vi "CoolLED_Control_v1.0.vi"(8 "error in":errorcluster) -> (0 "error out":errorcluster)   [LabVIEW 2025]
uses:
  SubVIs/States.ctl
  <vilib>/Instr/_visa.llb/VISA Configure Serial Port (Instr).vi
panel:
  in  "Tab Control":enum32{"Commands", "Expert"}(tab)
  in  "Presets":enum16{"DAPI", "GFP", "RFP", "None", "Multiple"}(ring)=enum."None"
  in  "Store":bool
  in  "Cluster":T1 {"Green-Red" step=1 scale=0.0..100.0; "Blue" step=1 scale=0.0..100.0; "Violet" step=1 scale=0.0..100.0}
  in  "VISA resource name":refnum<visa-resource-name>="COM5"
  out "Current command":string="CSSAXF000BXF000CXF000\r\n"
  in  "Stop":bool
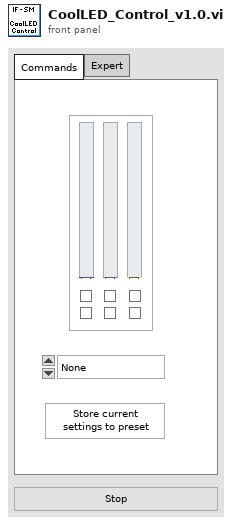
[diagram p1: front panel]
types:
  T1 = cluster{"Violet":u8, "Blue":u8, "Green-Red":u8, "A(S)Selected/(N)Unselected":bool, "B(S)Selected/(N)Unselected":bool, "C(S)Selected/(N)Unselected":bool, "A(N)ON/(F)OFF":bool, "(N)ON/(F)OFF":bool, "C(N)ON/(F)OFF":bool}
  T2 = typedef "States.ctl" = enum16{"Initialize", "Wait for Event", "Close", "Store", "Send", "Create_command", "Presets"}
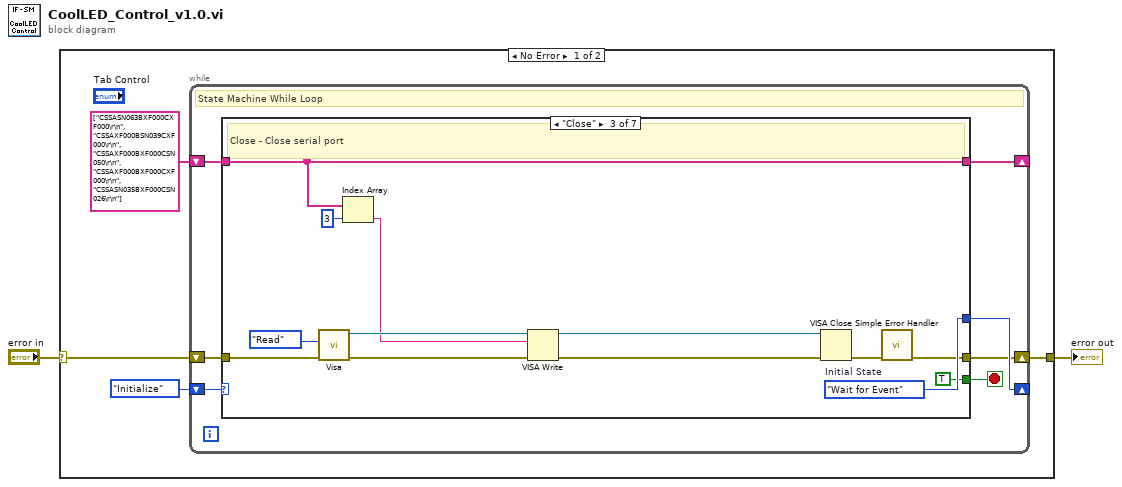
[diagram p0: block diagram]
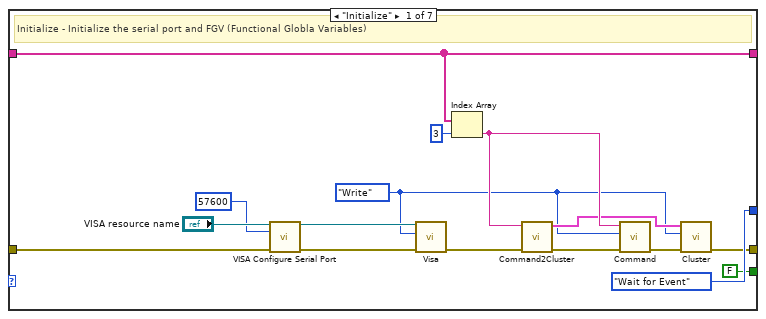
[diagram p2: hidden frame]
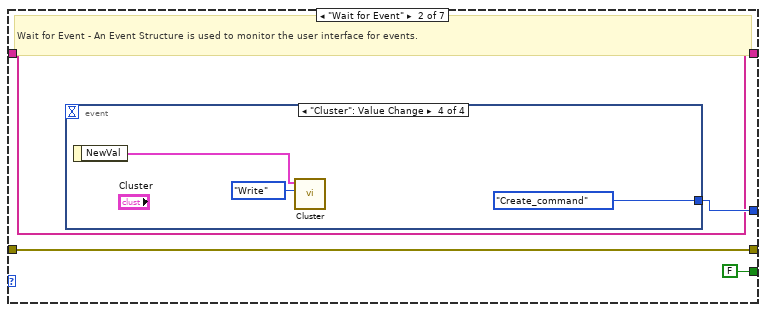
[diagram p3: hidden frame]
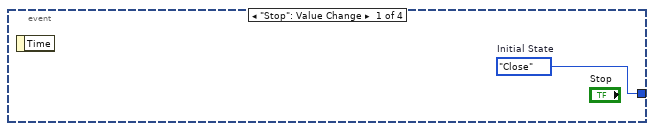
[diagram p4: hidden frame]
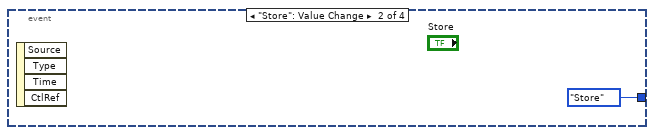
[diagram p5: hidden frame]
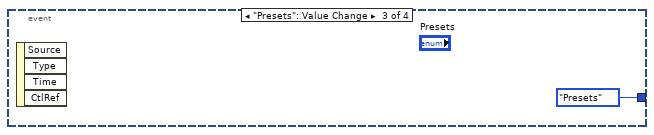
[diagram p6: hidden frame]
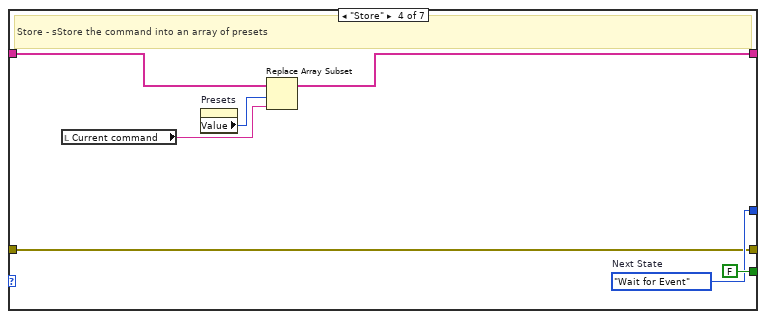
[diagram p7: hidden frame]
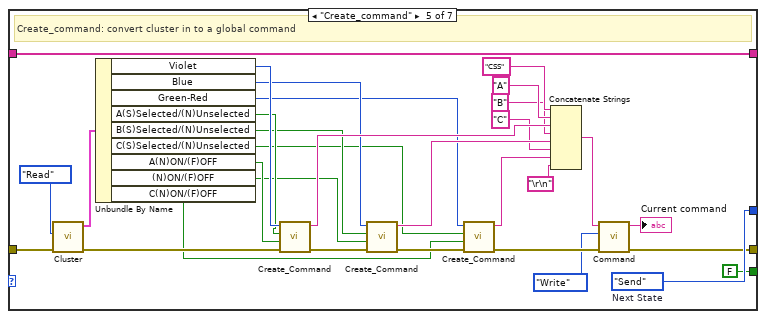
[diagram p8: hidden frame]
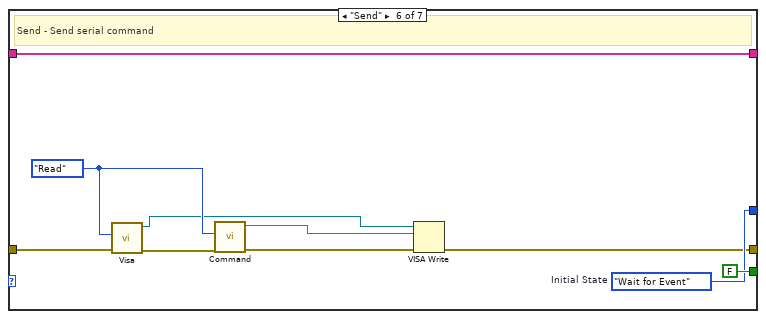
[diagram p9: hidden frame]
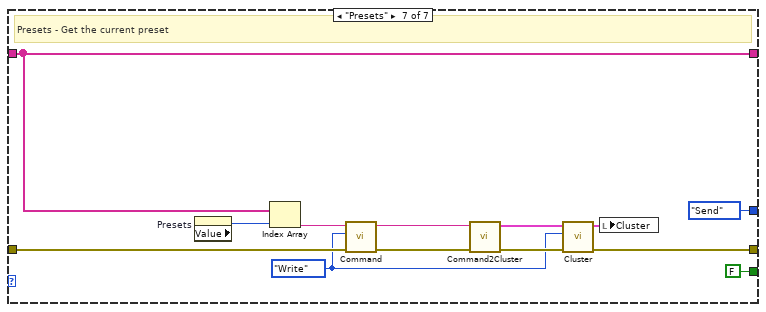
[diagram p10: hidden frame]
diagram:
  n1 = case shown="No Error" "error in" {
    selector: "error in" -> [w5 w114]
    tunnel: [w4 w114] -> w1
    frame No Error {
      n2 = while {
        shift-right: [w13] -> _
        shift-left: States."Initialize" ("Initial State") -> [w11]
        shift-right: [w9] -> w4
        shift-left: w5 -> [w10]
        shift-right: [w7] -> _
        shift-left: string[] ["CSSASN063BXF000CXF000\r\n", "CSSAXF000BSN039CXF000\r\n", "CSSAXF000BXF000CSN050\r\n", "CSSAXF000BXF000CXF000\r\n", "CSSASN035BXF000CSN026\r\n"] ("output array") -> [w8]
        stop <- w12 stop-if-true
        # "State Machine While Loop"
        n3 = case "State Machine Case Structure" shown="\"Close\"" w11 {
          tunnel: [States."Wait for Event" ("Initial State") w33 w52 w58 w90 w99 States."Send" ("Initial State")] -> w13
          tunnel: [FALSE ("Stop the Loop") FALSE ("Stop the Loop") TRUE ("Stop the Loop") FALSE ("Stop the Loop") FALSE ("Stop the Loop") FALSE ("Stop the Loop") FALSE ("Stop the Loop")] -> w12
          tunnel: w10 -> [w26 w31 w47 w57 w72 w94 w110]
          tunnel: [w16 w31 w49 w57 w74 w96 w103] -> w9
          tunnel: w8 -> [w21 w30 w42 w56 w79 w98 w108]
          tunnel: [w21 w30 w42 w53 w79 w98 w108] -> w7
          frame "Initialize" {
            w14 = enum16{"Write", "Read"}."Write" ("Action")
            # "Initialize - Initialize the serial port and FGV (Functional Globla Variables)"
            n4 = call-poly "VISA Configure Serial Port"("VISA resource name"="VISA resource name", "baud rate (9600)"=u32 57600, "error in (no error)"=w26) -> ("VISA resource name out"=w24:refnum<visa-resource-name>, "error out"=w23:errorcluster)  [unwired: 6 in, 5 out]
            n5 = call "Visa.vi"("error in"=w23, "Action"=w14, "VISA resource name"=w24) -> ("error out"=w22:errorcluster)  [unwired: 7 in, 1 out]
            n6 = Index Array(array=w21, index=3) -> (element=w19:string)
            n7 = call "Command2Cluster.vi"("error in"=w22, "Current command"=w19) -> ("error out"=w18:errorcluster, "Cluster"=w15:T1)  [unwired: 8 in]
            n8 = call "Command.vi"("error in"=w18, "Action"=w14, "Command"=w19) -> ("error out"=w17:errorcluster)  [unwired: 7 in, 1 out]
            n9 = call "Cluster.vi"("error in"=w17, "Action"=w14, "Cluster"=w15) -> ("error out"=w16:errorcluster)  [unwired: 7 in, 1 out]
          }
          frame "Wait for Event" {
            # "Wait for Event - An Event Structure is used to monitor the user interface for events."
            n10 = event shown="[3] \"Cluster\": Value Change" {
              selector: _ -> [_ _ _ _]
              dyn-events: _ -> [_ _ _ _]
              timeout: _ -> [_ _ _ _]
              tunnel: [w34 States."Store" ("Initial State") States."Presets" ("Initial State") States."Create_command" ("Initial State")] -> w33
              event "Stop": Value Change {
                w34 = States."Close"  # Initial State
                n11 = event-data() -> ()  [unwired: 1 in, 1 out]
              }
              event "Store": Value Change {
                n12 = event-data() -> ()  [unwired: 1 in, 4 out]
              }
              event "Presets": Value Change {
                n13 = event-data() -> ()  [unwired: 1 in, 4 out]
              }
              event "Cluster": Value Change {
                n14 = event-data() -> ("NewVal"=w38:T1)  [unwired: 1 in]
                n15 = call "Cluster.vi"("Action"=enum16{"Write", "Read"}."Write", "Cluster"=w38) -> ()  [unwired: 8 in, 2 out]
              }
            }
          }
          frame "Close" {
            w52 = States."Wait for Event"  # Initial State
            # "Close - Close serial port"
            n16 = call "Visa.vi"("error in"=w47, "Action"=enum16{"Write", "Read"}."Read") -> ("error out"=w46:errorcluster, "VISA resource name"=w44:refnum<visa-resource-name>)  [unwired: 8 in]
            n17 = Index Array(array=w42, index=3) -> (element=w40:string)
            n18 = VISA Write(VISA resource name=w44, write buffer=w40, error in (no error)=w46) -> (VISA resource name out=w43:refnum<visa-resource-name>, error out=w45:errorcluster)  [unwired: 1 out]
            n19 = VISA Close(VISA resource name=w43, error in (no error)=w45) -> (error out=w50:errorcluster)
            n20 = call <vilib>:"Simple Error Handler.vi"("error in (no error)"=w50) -> ("error out"=w49:errorcluster)  [unwired: 1 in, 7 out]
          }
          frame "Store" {
            w58 = States."Wait for Event"  # Next State
            # "Store - sStore the command into an array of presets"
            n21 = local read "Current command"() -> (w54:string)
            n22 = property on="Presets" class="Enum (strict)"() -> ("Value"=w55:enum16{"DAPI", "GFP", "RFP", "None", "Multiple"})  [unwired: 2 in, 2 out]
            n23 = Replace Array Subset(array=w56, new element=w54, index=w55) -> (w53:string[])
          }
          frame "Create_command" {
            w90 = States."Send"  # Next State
            # "Create_command: convert cluster in to a global command"
            n24 = call "Cluster.vi"("error in"=w72, "Action"=enum16{"Write", "Read"}."Read") -> ("error out"=w71:errorcluster, "Cluster"=w69:T1)  [unwired: 8 in]
            n25 = Unbundle By Name(w69) -> ("Violet"=w68:u8, "Blue"=w67:u8, "Green-Red"=w66:u8, "A(S)Selected/(N)Unselected"=w65:bool, "B(S)Selected/(N)Unselected"=w64:bool, "C(S)Selected/(N)Unselected"=w63:bool, "A(N)ON/(F)OFF"=w62:bool, "(N)ON/(F)OFF"=w61:bool, "C(N)ON/(F)OFF"=w60:bool)
            n26 = call "Create_Command.vi"("error in"=w71, "On/OFF"=w62, "Select"=w65, "Intensity"=w68) -> ("error out"=w88:errorcluster, "Command"=w84:string)  [unwired: 6 in]
            n27 = call "Create_Command.vi"("error in"=w88, "On/OFF"=w61, "Select"=w64, "Intensity"=w67) -> ("error out"=w87:errorcluster, "Command"=w82:string)  [unwired: 6 in]
            n28 = call "Create_Command.vi"("error in"=w87, "On/OFF"=w60, "Select"=w63, "Intensity"=w66) -> ("error out"=w77:errorcluster, "Command"=w80:string)  [unwired: 6 in]
            n29 = Concatenate Strings("CSS" ("string"), "A" ("string"), w84, "B" ("string"), w82, "C" ("string"), w80, "\r\n") -> (w76:string)
            n30 = call "Command.vi"("error in"=w77, "Action"=enum16{"Write", "Read"}."Write", "Command"=w76) -> ("error out"=w74:errorcluster, "Command"=→"Current command":string)  [unwired: 7 in]
          }
          frame "Send" {
            w92 = enum16{"Write", "Read"}."Read" ("Action")
            w99 = States."Wait for Event"  # Initial State
            # "Send - Send serial command"
            n31 = call "Visa.vi"("error in"=w94, "Action"=w92) -> ("error out"=w93:errorcluster, "VISA resource name"=w91:refnum<visa-resource-name>)  [unwired: 8 in]
            n32 = call "Command.vi"("error in"=w93, "Action"=w92) -> ("error out"=w97:errorcluster, "Command"=w95:string)  [unwired: 8 in]
            n33 = VISA Write(VISA resource name=w91, write buffer=w95, error in (no error)=w97) -> (error out=w96:errorcluster)  [unwired: 2 out]
          }
          frame "Presets" {
            w102 = enum16{"Write", "Read"}."Write" ("Action")
            # "Presets - Get the current preset"
            n34 = property on="Presets" class="Enum (strict)"() -> ("Value"=w111:enum16{"DAPI", "GFP", "RFP", "None", "Multiple"})  [unwired: 2 in, 2 out]
            n35 = Index Array(array=w108, index=w111) -> (element=w109:string)
            n36 = call "Command.vi"("error in"=w110, "Action"=w102, "Command"=w109) -> ("error out"=w104:errorcluster, "Command"=w107:string)  [unwired: 7 in]
            n37 = call "Command2Cluster.vi"("error in"=w104, "Current command"=w107) -> ("error out"=w105:errorcluster, "Cluster"=w106:T1)  [unwired: 8 in]
            n38 = call "Cluster.vi"("error in"=w105, "Action"=w102, "Cluster"=w106) -> ("error out"=w103:errorcluster, "Cluster"=w101:T1)  [unwired: 7 in]
            n39 = local write "Cluster"(w101) -> ()
          }
        }
      }
    }
    frame Error {
    }
  }
  "error out" <- w1
